vi "processCommandPublish.vi"(8 "error in (no error)":errorcluster, 11 "MiddlewareSALThisComponent in":refnum<class "MiddlewareSALThisComponent.lvclass">) -> (0 "error out":errorcluster, 3 "MiddlewareSALThisComponent out":refnum<class "MiddlewareSALThisComponent.lvclass">)   [LabVIEW 2016, in "MiddlewareSALThisComponent.lvclass"]
uses:
  MiddlewareSALThisComponent.lvclass
  home/andres/ct_cmpuserevents/ComponentTemplateCore/ComponentModel/ComponentModel/Middleware/Middleware.lvclass
  ComponentTemplateCore/ComponentModel/ComponentModel/Middleware/Middleware.lvclass/Middleware.ctl
  ComponentTemplateCore/ComponentModel/ComponentModel/MiddlewareProcessEvent/MiddlewareProcessEvent.lvclass/MiddlewareProcessEvent.ctl
  ComponentTemplateCore/ComponentModel/ComponentModel/CommandEvent/CommandEvent.lvclass/CommandEvent.ctl
  <vilib>/Utility/error.llb/DialogType.ctl
  ts_sallv_exa/DataTypes/logevent_InternalCommand.ctl
  ComponentTemplateCore/ComponentModel/ComponentModel/Middleware/Middleware.lvclass
  ComponentTemplateCore/ComponentModel/ComponentModel/CommandEvent/CommandEvent.lvclass
  ComponentTemplateCore/ComponentModel/ComponentModel/MiddlewareProcessEvent/MiddlewareProcessEvent.lvclass
  ts_sallv_exa/SALLV_EXA.lvlib
  ProgrammaticInitialization/ProgrammaticInitialization.lvclass
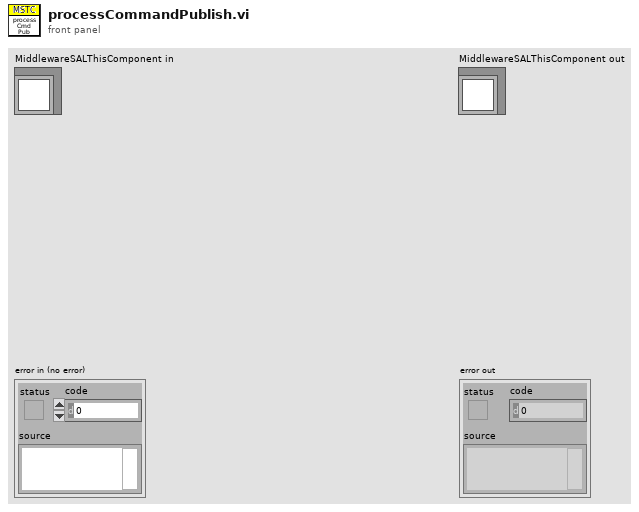
[diagram p1: front panel]
types:
  T1 = typedef "CommandEvents.ctl" = cluster{"command":refnum<user-event>}
  T2 = typedef "MiddlewareProcessEvents.ctl" = cluster{"disconnect":refnum<user-event>, "error":refnum<user-event>}
  T3 = typedef "SALLV_EXA.lvlib/logevent_InternalCommand.ctl" = cluster{"CommandObject[1000]":u8[], "priority":i32}
  T4 = typedef "DialogType.ctl" = u16
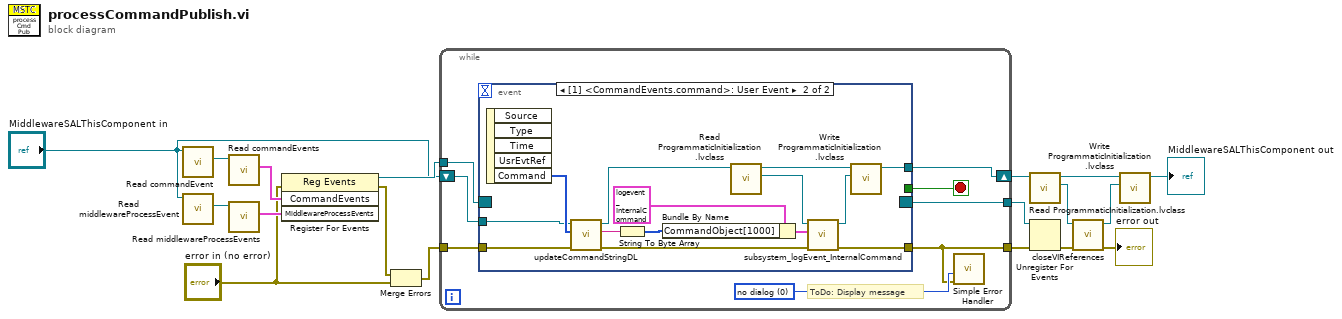
[diagram p0: block diagram]
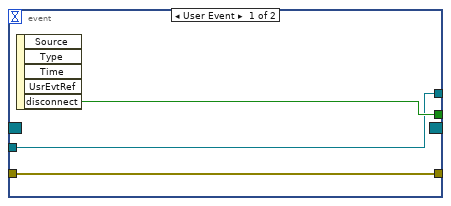
[diagram p2: hidden frame]
diagram:
  n1 = call "Read commandEvent.vi"("Middleware in"="MiddlewareSALThisComponent in") -> ("commandEvent"=w13:refnum<class "CommandEvent.lvclass">)  [unwired: 9 in, 1 out]
  n2 = call "Read middlewareProcessEvent.vi"("Middleware in"="MiddlewareSALThisComponent in") -> ("middlewareProcessEvent"=w12:refnum<class "MiddlewareProcessEvent.lvclass">)  [unwired: 9 in, 1 out]
  n3 = call "Read commandEvents.vi"("CommandEvent in"=w13) -> ("CommandEvents"=w10:T1)  [unwired: 9 in, 1 out]
  n4 = call "Read middlewareProcessEvents.vi"("MiddlewareProcessEvent in"=w12) -> ("MiddlewareProcessEvents"=w11:T2)  [unwired: 9 in, 1 out]
  n5 = register-events(error in="error in (no error)", w10, w11) -> (reference out=w18:refnum<event-registration>, error out=w16:errorcluster)  [unwired: 1 in]
  n6 = Merge Errors(w16, "error in (no error)") -> (w17:errorcluster)
  n7 = while {
    tunnel: w18 -> [w26]
    tunnel: [w23] -> w14
    tunnel: w17 -> [w22]
    tunnel: [w21] -> w15
    shift-right: [w19] -> w2
    shift-left: "MiddlewareSALThisComponent in" -> [w20]
    stop <- w25 stop-if-true
    w24 = T4 0 items=["no dialog", "OK message", "continue or stop message", "OK message + warnings", "continue/stop + warnings"] ("type of dialog (OK msg:1)")
    # "ToDo: Display message"
    n8 = event shown="[1] <CommandEvents.command>: User Event" {
      selector: w26 -> [_ _]
      dyn-events: [_ _] -> w21
      timeout: _ -> [_ _]
      tunnel: [w28 _] -> w25
      tunnel: [w29 w36] -> w23
      tunnel: w22 -> [w29 w43]
      tunnel: w20 -> [w27 w41]
      tunnel: [w27 w31] -> w19
      event User Event {
        n9 = event-data() -> ("disconnect"=w28:bool)  [unwired: 1 in, 4 out]
      }
      event User Event {
        n10 = event-data() -> ("Command"=w42:u8[])  [unwired: 1 in, 4 out]
        n11 = call "updateCommandStringDL.vi"("error in (no error)"=w43, "Command U8 Array"=w42, "MiddlewareSALThisComponent in"=w41) -> ("error out"=w35:errorcluster, "Cmd str"=w40:string, "MiddlewareSALThisComponent out"=w37:refnum<class "MiddlewareSALThisComponent.lvclass">)  [unwired: 6 in]
        n12 = String To Byte Array(string=w40) -> (unsigned byte array=w38:u8[])
        n13 = Bundle By Name(cluster=T3 {"CommandObject[1000]"=[0, 0, 0, 0, 0, 0, 0, 0, 0, 0, 0, 0, 0, 0, 0, 0, 0, 0, 0, 0, 0, 0, 0, 0, 0, 0, 0, 0, 0, 0, 0, 0, 0, 0, 0, 0, 0, 0, 0, 0, 0, 0, 0, 0, 0, 0, 0, 0, 0, 0, 0, 0, 0, 0, 0, 0, 0, 0, 0, 0, 0, 0, 0, 0, 0, 0, 0, 0, 0, 0, 0, 0, 0, 0, 0, 0, 0, 0, 0, 0, 0, 0, 0, 0, 0, 0, 0, 0, 0, 0, 0, 0, 0, 0, 0, 0, 0, 0, 0, 0, 0, 0, 0, 0, 0, 0, 0, 0, 0, 0, 0, 0, 0, 0, 0, 0, 0, 0, 0, 0, 0, 0, 0, 0, 0, 0, 0, 0, 0, 0, 0, 0, 0, 0, 0, 0, 0, 0, 0, 0, 0, 0, 0, 0, 0, 0, 0, 0, 0, 0, 0, 0, 0, 0, 0, 0, 0, 0, 0, 0, 0, 0, 0, 0, 0, 0, 0, 0, 0, 0, 0, 0, 0, 0, 0, 0, 0, 0, 0, 0, 0, 0, 0, 0, 0, 0, 0, 0, 0, 0, 0, 0, 0, 0, 0, 0, 0, 0, 0, 0, 0, 0, 0, 0, 0, 0, 0, 0, 0, 0, 0, 0, 0, 0, 0, 0, 0, 0, 0, 0, 0, 0, 0, 0, 0, 0, 0, 0, 0, 0, 0, 0, 0, 0, 0, 0, 0, 0, 0, 0, 0, 0, 0, 0, 0, 0, 0, 0, 0, 0, 0, 0, 0, 0, 0, 0, 0, 0, 0, 0, 0, 0, 0, 0, 0, 0, 0, 0, 0, 0, 0, 0, 0, 0, 0, 0, 0, 0, 0, 0, 0, 0, 0, 0, 0, 0, 0, 0, 0, 0, 0, 0, 0, 0, 0, 0, 0, 0, 0, 0, 0, 0, 0, 0, 0, 0, 0, 0, 0, 0, 0, 0, 0, 0, 0, 0, 0, 0, 0, 0, 0, 0, 0, 0, 0, 0, 0, 0, 0, 0, 0, 0, 0, 0, 0, 0, 0, 0, 0, 0, 0, 0, 0, 0, 0, 0, 0, 0, 0, 0, 0, 0, 0, 0, 0, 0, 0, 0, 0, 0, 0, 0, 0, 0, 0, 0, 0, 0, 0, 0, 0, 0, 0, 0, 0, 0, 0, 0, 0, 0, 0, 0, 0, 0, 0, 0, 0, 0, 0, 0, 0, 0, 0, 0, 0, 0, 0, 0, 0, 0, 0, 0, 0, 0, 0, 0, 0, 0, 0, 0, 0, 0, 0, 0, 0, 0, 0, 0, 0, 0, 0, 0, 0, 0, 0, 0, 0, 0, 0, 0, 0, 0, 0, 0, 0, 0, 0, 0, 0, 0, 0, 0, 0, 0, 0, 0, 0, 0, 0, 0, 0, 0, 0, 0, 0, 0, 0, 0, 0, 0, 0, 0, 0, 0, 0, 0, 0, 0, 0, 0, 0, 0, 0, 0, 0, 0, 0, 0, 0, 0, 0, 0, 0, 0, 0, 0, 0, 0, 0, 0, 0, 0, 0, 0, 0, 0, 0, 0, 0, 0, 0, 0, 0, 0, 0, 0, 0, 0, 0, 0, 0, 0, 0, 0, 0, 0, 0, 0, 0, 0, 0, 0, 0, 0, 0, 0, 0, 0, 0, 0, 0, 0, 0, 0, 0, 0, 0, 0, 0, 0, 0, 0, 0, 0, 0, 0, 0, 0, 0, 0, 0, 0, 0, 0, 0, 0, 0, 0, 0, 0, 0, 0, 0, 0, 0, 0, 0, 0, 0, 0, 0, 0, 0, 0, 0, 0, 0, 0, 0, 0, 0, 0, 0, 0, 0, 0, 0, 0, 0, 0, 0, 0, 0, 0, 0, 0, 0, 0, 0, 0, 0, 0, 0, 0, 0, 0, 0, 0, 0, 0, 0, 0, 0, 0, 0, 0, 0, 0, 0, 0, 0, 0, 0, 0, 0, 0, 0, 0, 0, 0, 0, 0, 0, 0, 0, 0, 0, 0, 0, 0, 0, 0, 0, 0, 0, 0, 0, 0, 0, 0, 0, 0, 0, 0, 0, 0, 0, 0, 0, 0, 0, 0, 0, 0, 0, 0, 0, 0, 0, 0, 0, 0, 0, 0, 0, 0, 0, 0, 0, 0, 0, 0, 0, 0, 0, 0, 0, 0, 0, 0, 0, 0, 0, 0, 0, 0, 0, 0, 0, 0, 0, 0, 0, 0, 0, 0, 0, 0, 0, 0, 0, 0, 0, 0, 0, 0, 0, 0, 0, 0, 0, 0, 0, 0, 0, 0, 0, 0, 0, 0, 0, 0, 0, 0, 0, 0, 0, 0, 0, 0, 0, 0, 0, 0, 0, 0, 0, 0, 0, 0, 0, 0, 0, 0, 0, 0, 0, 0, 0, 0, 0, 0, 0, 0, 0, 0, 0, 0, 0, 0, 0, 0, 0, 0, 0, 0, 0, 0, 0, 0, 0, 0, 0, 0, 0, 0, 0, 0, 0, 0, 0, 0, 0, 0, 0, 0, 0, 0, 0, 0, 0, 0, 0, 0, 0, 0, 0, 0, 0, 0, 0, 0, 0, 0, 0, 0, 0, 0, 0, 0, 0, 0, 0, 0, 0, 0, 0, 0, 0, 0, 0, 0, 0, 0, 0, 0, 0, 0, 0, 0, 0, 0, 0, 0, 0, 0, 0, 0, 0, 0, 0, 0, 0, 0, 0, 0, 0, 0, 0, 0, 0, 0, 0, 0, 0, 0, 0, 0, 0, 0, 0, 0, 0, 0, 0, 0, 0, 0, 0, 0, 0, 0, 0, 0, 0, 0, 0, 0, 0, 0, 0, 0, 0, 0, 0, 0, 0, 0, 0, 0, 0, 0, 0, 0, 0, 0, 0, 0, 0, 0, 0, 0, 0, 0, 0, 0, 0, 0, 0, 0, 0, 0, 0, 0, 0, 0, 0, 0, 0, 0, 0, 0, 0, 0, 0, 0, 0, 0, 0, 0, 0, 0, 0, 0, 0, 0, 0, 0, 0, 0, 0, 0, 0, 0, 0, 0, 0, 0, 0, 0, 0, 0, 0, 0, 0, 0, 0, 0, 0, 0, 0, 0, 0, 0, 0, 0, 0, 0, 0, 0, 0, 0, 0, 0, 0, 0, 0, 0, 0, 0, 0, 0, 0, 0, 0, 0, 0, 0, 0, 0], "priority"=0} ("logevent_InternalCommand_Ctl"), "CommandObject[1000]"=w38) -> (w34:T3)
        n14 = call-dynamic "Read ProgrammaticInitialization.lvclass.vi"("MiddlewareSALThisComponent in"=w37) -> ("ProgrammaticInitialization.lvclass"=w33:refnum<class "ProgrammaticInitialization.lvclass">, "MiddlewareSALThisComponent out"=w32:refnum<class "MiddlewareSALThisComponent.lvclass">)  [unwired: 8 in, 1 out]
        n15 = call "subsystem_logEvent_InternalCommand.vi"("error in (no error)"=w35, "logevent_InternalCommand in"=w34, "ProgrammaticInitialization in"=w33) -> ("error out"=w36:errorcluster, "ProgrammaticInitialization out"=w30:refnum<class "ProgrammaticInitialization.lvclass">)  [unwired: 6 in, 1 out]
        n16 = call-dynamic "Write ProgrammaticInitialization.lvclass.vi"("ProgrammaticInitialization.lvclass"=w30, "MiddlewareSALThisComponent in"=w32) -> ("MiddlewareSALThisComponent out"=w31:refnum<class "MiddlewareSALThisComponent.lvclass">)  [unwired: 8 in, 1 out]
      }
    }
    n17 = call <vilib>:"Simple Error Handler.vi"("type of dialog (OK msg:1)"=w24, "error in (no error)"=w23) -> ()  [unwired: 3 in, 5 out]
  }
  n18 = call-dynamic "Read ProgrammaticInitialization.lvclass.vi"("MiddlewareSALThisComponent in"=w2) -> ("ProgrammaticInitialization.lvclass"=w7:refnum<class "ProgrammaticInitialization.lvclass">, "MiddlewareSALThisComponent out"=w6:refnum<class "MiddlewareSALThisComponent.lvclass">)  [unwired: 8 in, 1 out]
  n19 = Unregister For Events(event registration refnum=w15, error in=w14) -> (error out=w4:errorcluster)
  n20 = call "closeVIReferences.vi"("error in (no error)"=w4, "ProgrammaticInitialization in"=w7) -> ("error out"=→"error out":errorcluster, "ProgrammaticInitialization out"=w5:refnum<class "ProgrammaticInitialization.lvclass">)  [unwired: 8 in]
  n21 = call-dynamic "Write ProgrammaticInitialization.lvclass.vi"("ProgrammaticInitialization.lvclass"=w5, "MiddlewareSALThisComponent in"=w6) -> ("MiddlewareSALThisComponent out"=→"MiddlewareSALThisComponent out":refnum<class "MiddlewareSALThisComponent.lvclass">)  [unwired: 8 in, 1 out]
